vi "Pic Unflatten RGBA Pixmap.vi"(8 "error in (no error)":errorcluster, 10 "BG Color":u32(colorbox), 11 "32-bit image data (ARGB)":T1) -> (0 "error out":errorcluster, 3 "24-bit pixmap":u32[][](array[numeric]) format="%x")   [LabVIEW 2018, in "Picture Process.lvclass"]
doc: "Converts a cluster of image data into a 2D array."
uses:
  Picture Process.lvclass
  <vilib>/picture/picture.llb/imagedata.ctl
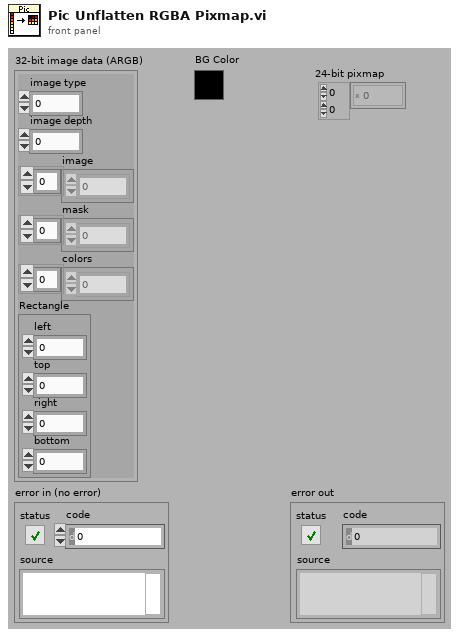
[diagram p1: front panel]
types:
  T1 = typedef "imagedata.ctl" = cluster{"image type":i32, "image depth":i32, "image":u8[], "mask":u8[], "colors":u32[], "Rectangle":cluster{"left":i16, "top":i16, "right":i16, "bottom":i16}}
  T2 = cluster{"left":i16, "top":i16, "right":i16, "bottom":i16}
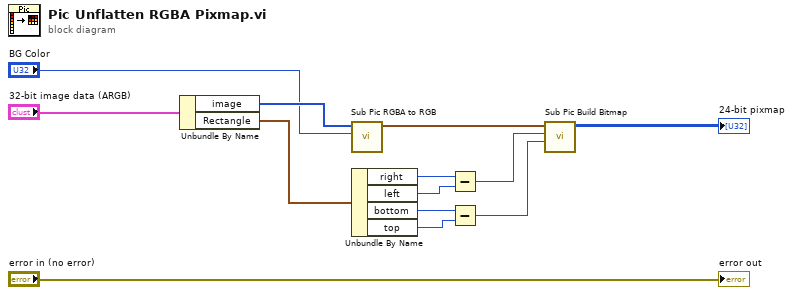
[diagram p0: block diagram]
diagram:
  n1 = Unbundle By Name("32-bit image data (ARGB)") -> ("image"=w3:u8[], "Rectangle"=w12:T2)
  n2 = call "Sub Pic RGBA to RGB.vi"("Default Color"="BG Color", "RGBA Array"=w3) -> ("RGB Array"=w10:cluster{"R":u8, "G":u8, "B":u8}[])  [unwired: 9 in]
  n3 = Unbundle By Name(w12) -> ("right"=w9:i16, "left"=w8:i16, "bottom"=w7:i16, "top"=w6:i16)
  n4 = Subtract(x=w9, y=w8) -> (x-y=w5:i16)
  n5 = Subtract(x=w7, y=w6) -> (x-y=w4:i16)
  n6 = call "Sub Pic Build Bitmap.vi"("Height"=w4, "Width"=w5, "RGB Array"=w10) -> ("24-bit pixmap (RGB)"=→"24-bit pixmap":u32[][])  [unwired: 8 in]
  "error out" <- "error in (no error)"
